vi "set switch.vi"(8 "error in (no error)":errorcluster, 9 "state":bool, 10 "channel":dbl, 11 "Agilent 34980A in":refnum<class "Agilent 34980A.lvclass">) -> (0 "error out":errorcluster, 3 "Agilent 34980A out":refnum<class "Agilent 34980A.lvclass">)   [LabVIEW 2017, in "Agilent 34980A.lvclass"]
doc: "Agilent:\nset a switch of \"channel\" to \"state\""
uses:
  Agilent 34980A.lvclass
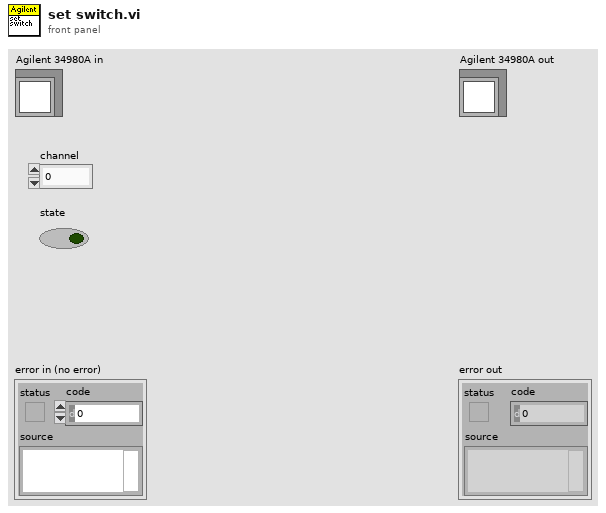
[diagram p1: front panel]
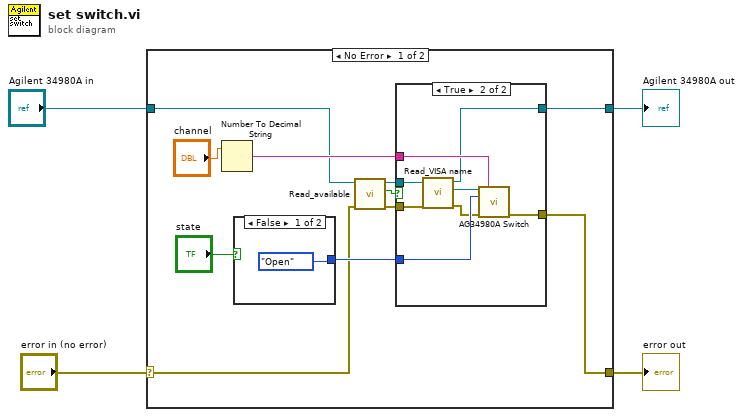
[diagram p0: block diagram]
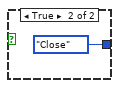
[diagram p3: hidden frame]
diagram:
  n1 = case shown="No Error" "error in (no error)" {
    selector: "error in (no error)" -> [w7 w29]
    tunnel: [w15 w29] -> w3
    tunnel: [w8 w28] -> w1
    tunnel: "Agilent 34980A in" -> [w10 w28]
    frame No Error {
      n2 = Number To Decimal String(number="channel") -> (decimal integer string=w11:string)  [unwired: 1 in]
      n3 = case shown="False" "state" {
        tunnel: [enum16{"Close", "Open"}."Open" ("Open/Close (0:Close)") enum16{"Close", "Open"}."Close" ("Open/Close (0:Close)")] -> w13
        frame False {
        }
        frame True {
        }
      }
      n4 = call-dynamic "Read_available.vi"("error in (no error)"=w7, "instrument in"=w10) -> ("error out"=w5:errorcluster, "available?"=w6:bool, "instrument out"=w9:refnum<class "Agilent 34980A.lvclass">)  [unwired: 7 in]
      n5 = case shown="True" w6 {
        tunnel: [w17 w25] -> w15
        tunnel: w13 -> [_ w23]
        tunnel: w11 -> [_ w22]
        tunnel: w9 -> [w16 w20]
        tunnel: [w16 w19] -> w8
        tunnel: w5 -> [w17 w18]
        frame False {
        }
        frame True {
          n6 = call-dynamic "Read_VISA name.vi"("error in (no error)"=w18, "instrument in"=w20) -> ("error out"=w21:errorcluster, "VISA resource name"=w24:refnum<visa-resource-name>, "instrument out"=w19:refnum<class "Agilent 34980A.lvclass">)  [unwired: 7 in]
          n7 = call "AG34980A Switch.vi"("VISA resource name"=w24, "Channel List"=w22, "Open/Close (0:Close)"=w23, "error in (no error)"=w21) -> ("error out"=w25:errorcluster)  [unwired: 9 in, 2 out]
        }
      }
    }
    frame Error {
    }
  }
  "error out" <- w3
  "Agilent 34980A out" <- w1
